vi "Named_Serial_Comms.vi"(0 "Channel Name":string, 1 "Write String":string, 2 "Timeout/ms":u32=500, 4 "!Error retries":i32=10, 6 "!Timeout retries":i32=3, 9 "Port Name":string, 11 "Term Grep":string="\r$", 12 "Log Errors?":bool=TRUE, 13 "Terminate Count":i32) -> (3 "Read":string="This is simulation mode", 10 "millisecond timer value":u32, 14 "Timed out":bool, 15 "Serial Error":bool)   [LabVIEW 2015]
doc: "The Serial Communication VI performs bidirectional communication with a port. It initializes the port, writes a string to the port, and performs a read with timeout. The Read with Timeout will wait until a terminating character is received or the time limit is up, whichever comes first.\nThe initialisation parameters, terminating character, and timeout, are all set in the Serial Setup Global."
uses:
  Port_Params.ctl
  <vilib>/Instr/_visa.llb/VISA Find Search Mode.ctl
  <vilib>/Instr/serial.llb/serpConfig.vi
panel:
  out "Buffer Trash":string
  out "Terminated?":bool
  out "Error Description":string
  in  "Uppercase?":bool
  in  "Append Return?":bool
  in  "Force setup reload":bool
  in  "Save Setups?":bool
  in  "!stop":bool
  out "byte count":u32
  out "Port Initialised?":bool[](array[boolean])
  out "Setting Number":i32
  out "Ports having file settings":string[](array[string])
  out "enumerated ports":string[](array[string])
  out "load setups error":bool
  out "Audit trail":string[](array[string])=["Start", "Simulate"]
  out "Close Port error":i32
  out "read error code":i32
  out "n-bytes error code":i32
  out "Write error":i32
  out "Port Initialisation Parameters":T1={"Name"="", "flow control etc."={"input XON/XOFF"=FALSE, "input HW Handshake"=FALSE, "input alt HW HShk"=FALSE, "output XON/XOFF"=FALSE, "output HW Handshake"=FALSE, "output alt HW HShk"=FALSE, "XOFF byte "=0, "XON byte"=0, "parity err byte"=0}, "buffer size"=0, "baud rate"=9600, "data bits"=8, "stop bits"=enum."1 bit", "parity"=enum."no parity"} {"flow control etc."."parity err byte" format="%.0x"; "flow control etc."."XON byte" format="%.0x"; "flow control etc."."XOFF byte" format="%.0x"; "data bits" min=5 max=8 step=1}
  out "Initialise error":i32
  out "Port Settings Array":T1[](array[typedef]) {"flow control etc."."parity err byte" format="%.0x"; "flow control etc."."XON byte" format="%.0x"; "flow control etc."."XOFF byte" format="%.0x"; "data bits" min=5 max=8 step=1}
  out "Case":string="Simulate"
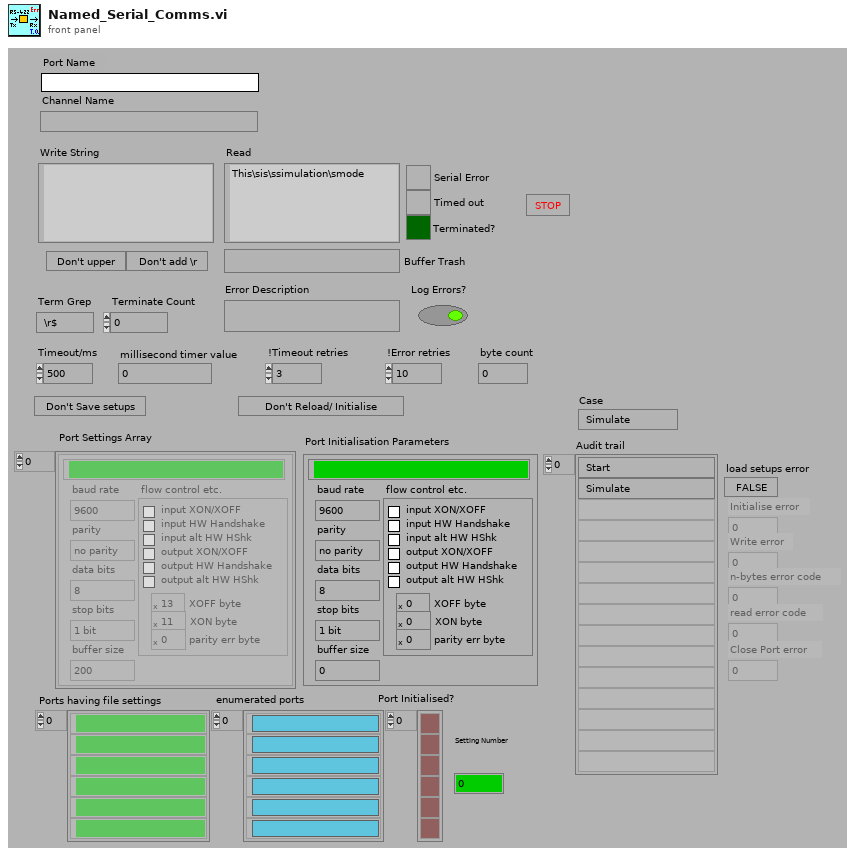
[diagram p1: front panel]
types:
  T1 = typedef "Port_Params.ctl" = cluster{"Name":string, "flow control etc.":cluster{"input XON/XOFF":bool, "input HW Handshake":bool, "input alt HW HShk":bool, "output XON/XOFF":bool, "output HW Handshake":bool, "output alt HW HShk":bool, "XOFF byte ":u8, "XON byte":u8, "parity err byte":u16}, "buffer size":u16, "baud rate":u32, "data bits":u16, "stop bits":enum16{"1 bit", "1.5 bits", "2 bits"}, "parity":enum16{"no parity", "odd parity", "even parity", "mark parity", "space parity"}}
  T2 = typedef "VISA Find Search Mode.ctl" = u32
  T3 = cluster{"input XON/XOFF":bool, "input HW Handshake":bool, "input alt HW HShk":bool, "output XON/XOFF":bool, "output HW Handshake":bool, "output alt HW HShk":bool, "XOFF byte ":u8, "XON byte":u8, "parity err byte":u16}
  T4 = enum16{"no parity", "odd parity", "even parity", "mark parity", "space parity"}
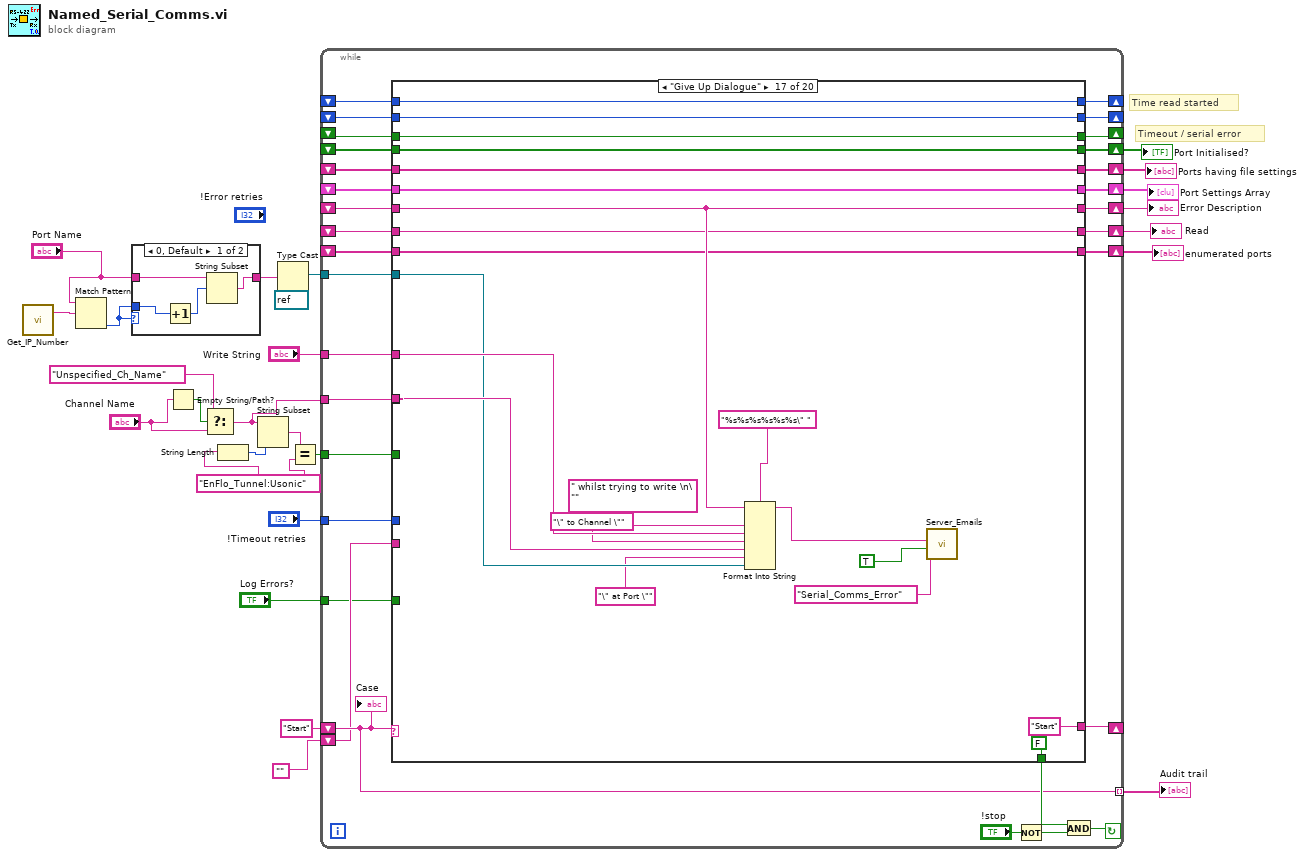
[diagram p0: block diagram]
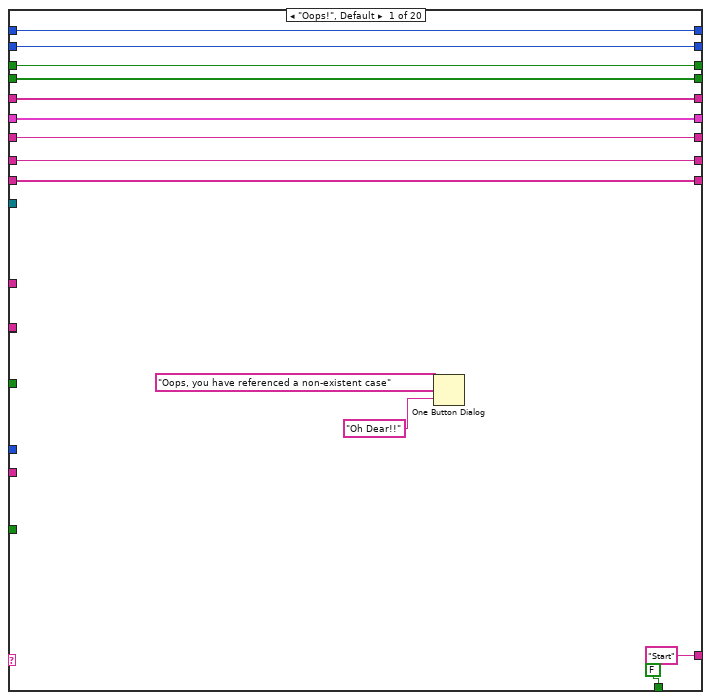
[diagram p3: hidden frame]
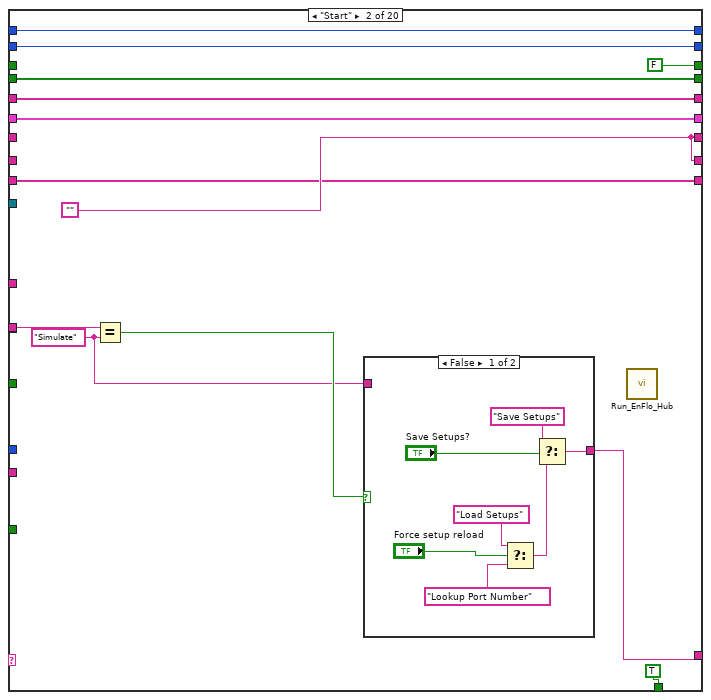
[diagram p4: hidden frame]
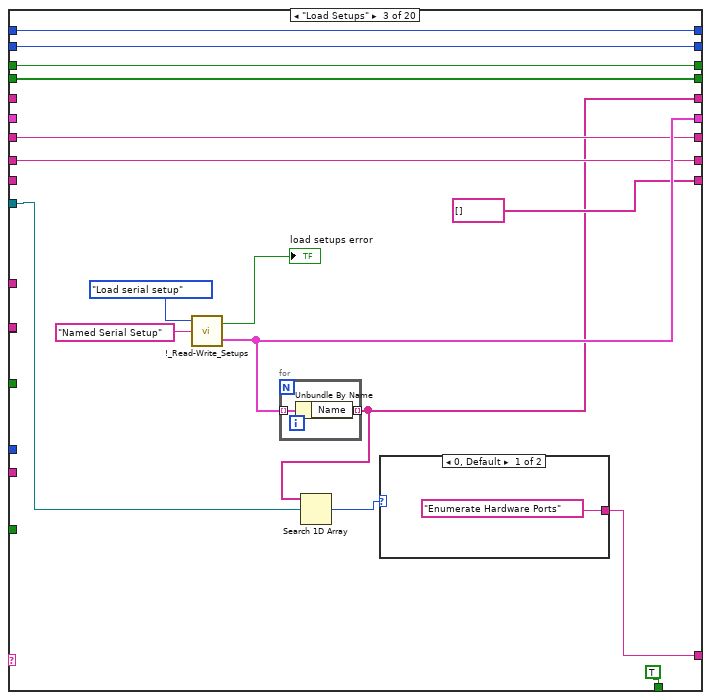
[diagram p6: hidden frame]
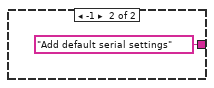
[diagram p7: hidden frame]
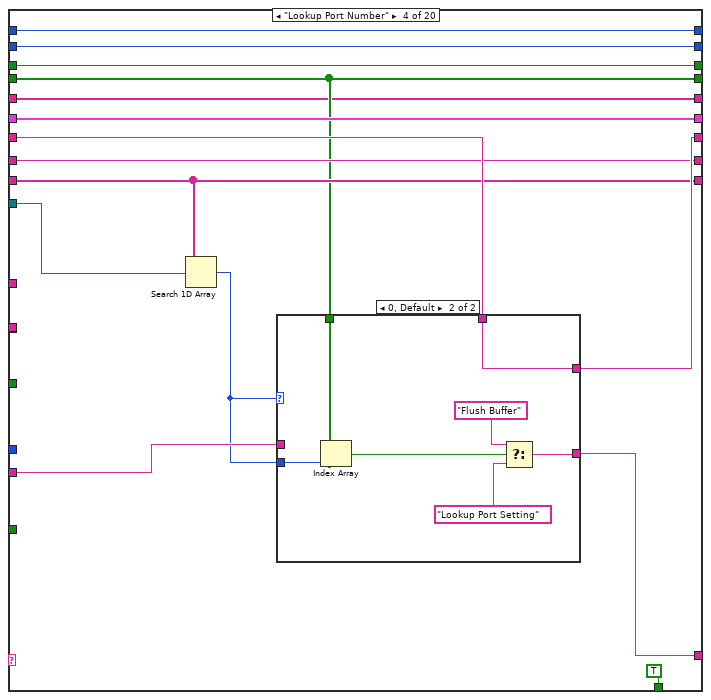
[diagram p8: hidden frame]
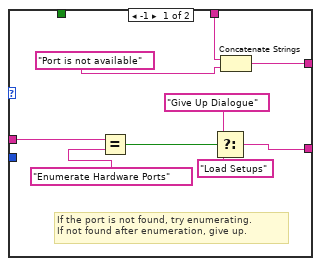
[diagram p9: hidden frame]
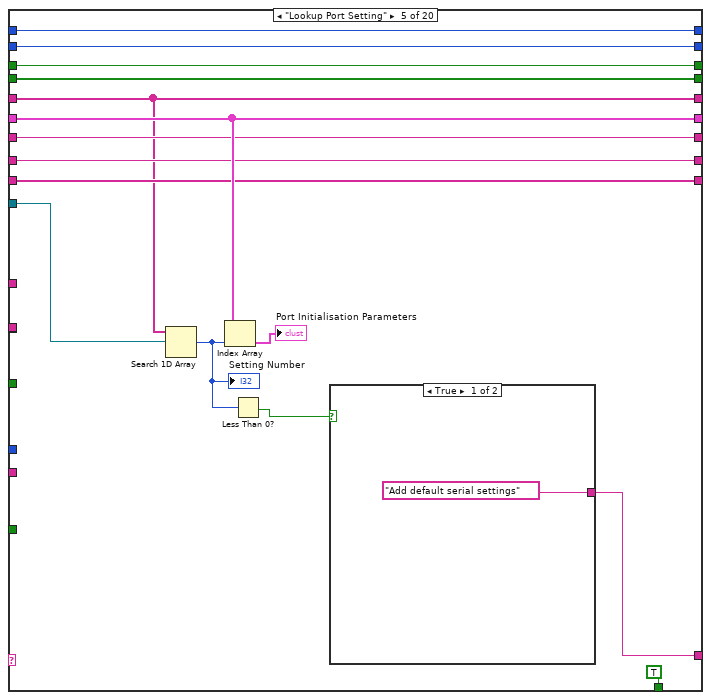
[diagram p10: hidden frame]
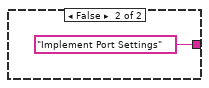
[diagram p11: hidden frame]
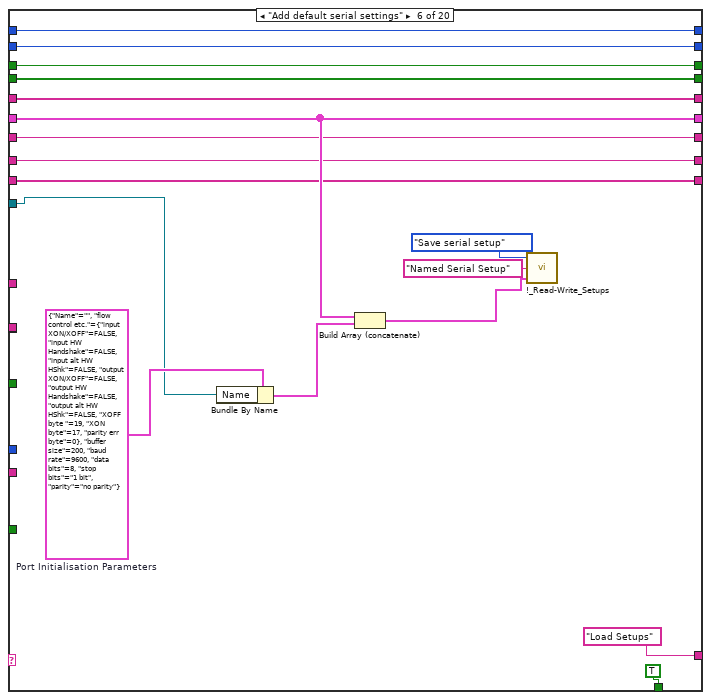
[diagram p12: hidden frame]
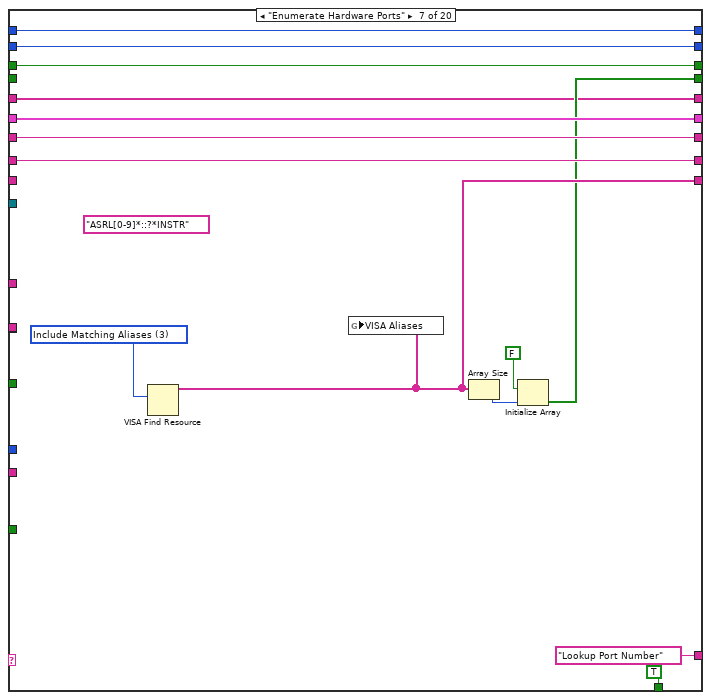
[diagram p13: hidden frame]
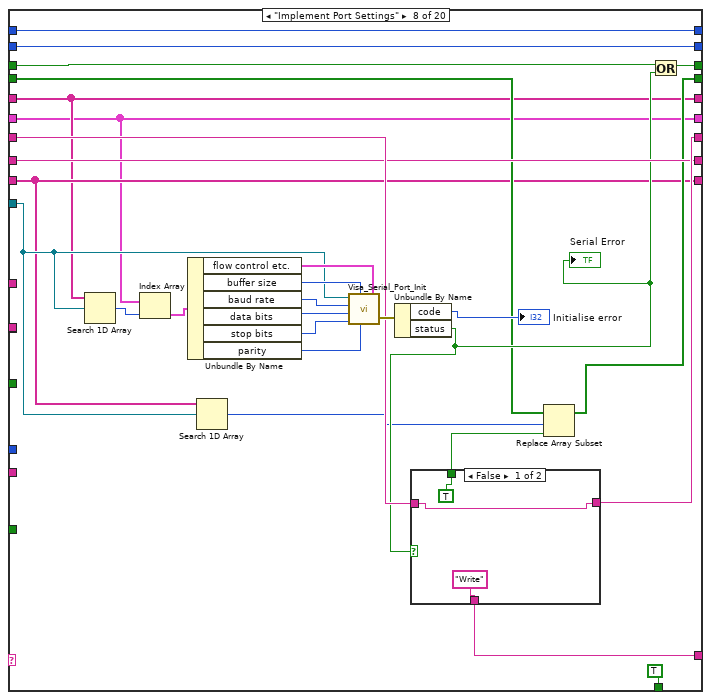
[diagram p14: hidden frame]
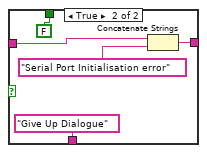
[diagram p15: hidden frame]
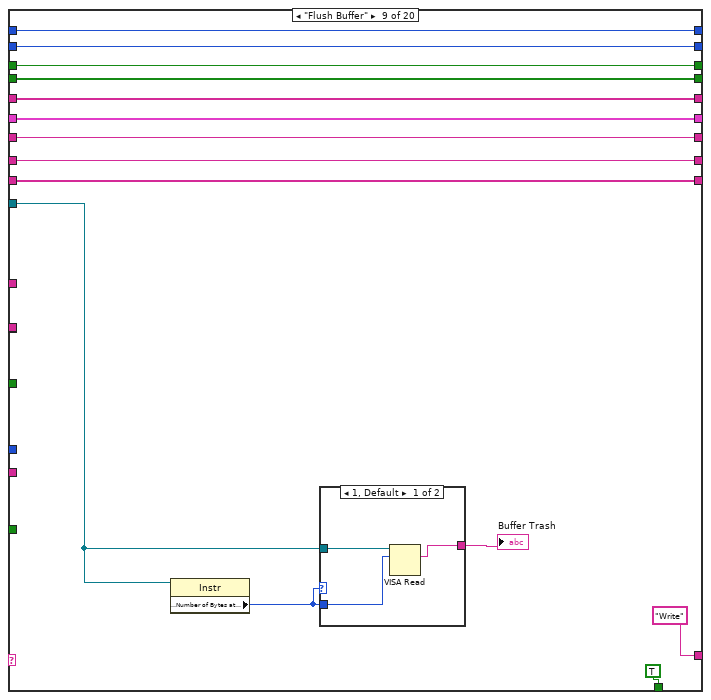
[diagram p16: hidden frame]
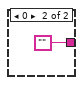
[diagram p17: hidden frame]
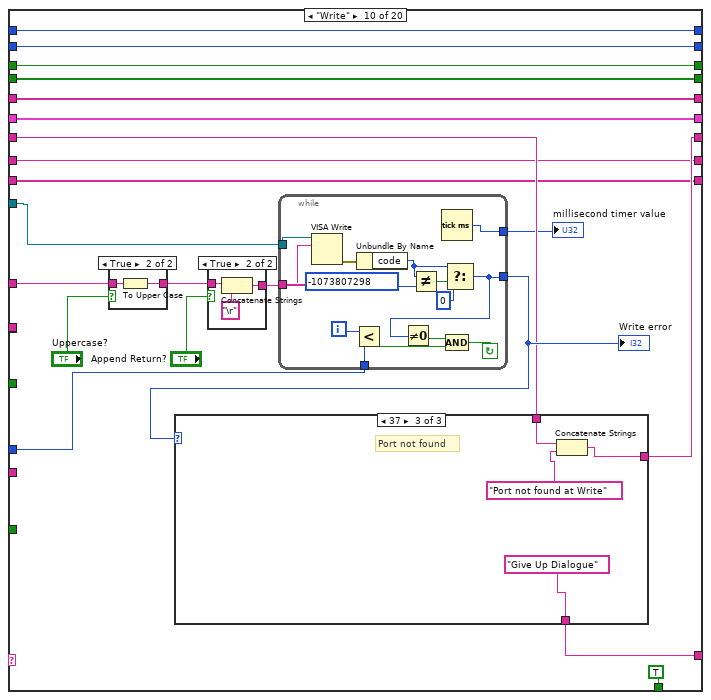
[diagram p18: hidden frame]
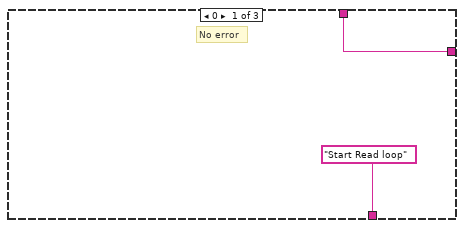
[diagram p19: hidden frame]
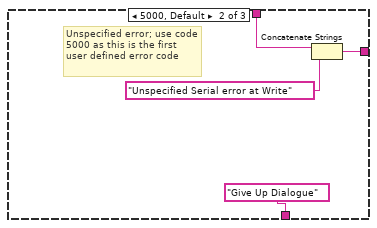
[diagram p20: hidden frame]
diagram:
  w19 = "EnFlo_Tunnel:Usonic"
  # "Time read started"
  # "Timeout / serial error"
  n1 = call "Get_IP_Number.vi"() -> ("IP Number"=w14:string)  [unwired: 1 out]
  n2 = Match Pattern(string="Port Name", regular expression=w14) -> (offset past match=w15:i32)  [unwired: 4 out]
  n3 = case shown="0, Default" w15 {
    tunnel: [w27 w31] -> w12
    tunnel: "Port Name" -> [w28 w31]
    tunnel: w15 -> [w30 _]
    frame 0, Default {
      n4 = Increment(x=w30) -> (x+1=w29:i32)
      n5 = String Subset(string=w28, offset (0)=w29) -> (substring=w27:string)  [unwired: 1 out]
    }
    frame -1 {
    }
  }
  n6 = Empty String/Path?(string/path="Channel Name") -> (empty?=w10:bool)
  n7 = Select(t="Unspecified_Ch_Name", s=w10, f="Channel Name") -> (s? t:f=w9:string)
  n8 = String Length(string=w19) -> (length=w21:i32)
  n9 = String Subset(string=w9, length (rest)=w21) -> (substring=w20:string)  [unwired: 1 out]
  n10 = Type Cast(type=refnum<visa-resource-name> refnum ("dup VISA resource name"), x=w12) -> (*(type *) &x=w17:refnum<visa-resource-name>)
  n11 = Equal?(x=w20, y=w19) -> (x = y?=w18:bool)
  n12 = while {
    tunnel: "!Timeout retries" -> [w52]
    tunnel: w9 -> [w54]
    shift-left: "" -> [w53]
    tunnel: [w55] -> w24 mode=indexing
    shift-left: "Start" -> [w55]
    shift-right: [w56] -> _
    tunnel: "Write String" -> [w61]
    tunnel: w17 -> [w62]
    tunnel: w18 -> [w51]
    tunnel: "Log Errors?" -> [w50]
    shift-right: [w49] -> w6
    shift-left: _ -> [w48]
    shift-right: [w46] -> w5
    shift-left: _ -> [w47]
    shift-right: [w45] -> w4
    shift-left: _ -> [w44]
    shift-right: [w43] -> w3
    shift-left: _ -> [w42]
    shift-right: [w41] -> _
    shift-left: _ -> [w40]
    shift-right: [w39] -> w2
    shift-left: _ -> [w38]
    shift-right: [w36] -> w1
    shift-left: _ -> [w37]
    shift-right: [w33] -> _
    shift-left: _ -> [w32]
    shift-right: [w35] -> _
    shift-left: _ -> [w34]
    stop <- w59 continue-if-true
    n13 = case shown="\"Give Up Dialogue\"" w55 {
      tunnel: w62 -> [_ _ w107 w131 w162 w179 _ w202 w238 w261 _ w322 w347 _ _ w440 w457 _ _ _]
      tunnel: w61 -> [_ _ _ _ _ _ _ _ _ w267 _ _ _ _ _ w433 w460 _ _ _]
      tunnel: ["Start" ("f") w88 w109 w129 w159 "Load Setups" ("f") "Lookup Port Number" w216 "Write" ("f") w264 "Bytes At Serial Port?" ("f") w324 w364 w387 w426 "Start" "Start" "Start" "Start" ("f") "Load Setups" ("f")] -> w56
      tunnel: [FALSE TRUE TRUE TRUE TRUE TRUE TRUE TRUE TRUE TRUE TRUE TRUE TRUE TRUE TRUE FALSE FALSE TRUE FALSE TRUE] -> w60
      tunnel: w54 -> [_ w86 _ _ _ _ _ _ _ _ _ _ _ _ _ w441 _ _ _ _]
      tunnel: w54 -> [_ _ _ _ _ _ _ _ _ _ _ _ _ _ _ _ w458 _ _ _]
      tunnel: w53 -> [_ _ _ w128 _ _ _ _ _ _ _ _ _ _ _ _ _ _ _ _]
      tunnel: w52 -> [_ _ _ _ _ _ _ _ _ w262 _ w323 _ _ _ _ _ _ _ _]
      tunnel: w51 -> [_ _ _ _ _ _ _ _ _ _ _ _ w360 _ _ _ _ _ _ _]
      tunnel: w50 -> [_ _ _ _ _ _ _ _ _ _ _ _ _ _ _ w439 _ _ _ _]
      tunnel: [w71 w83 w105 w127 w156 w173 w191 w199 w243 w260 w310 w321 w355 w380 w421 w438 w455 w473 w487 w498] -> w49
      tunnel: w48 -> [w71 w83 _ w127 w156 w173 w191 w199 w243 w260 w310 w321 w355 w380 w421 w438 w455 w473 w487 w498]
      tunnel: w47 -> [w70 _ w104 w126 w155 w172 w190 w211 w242 w258 w309 w320 w354 w379 w420 w437 w454 w472 w486 w497]
      tunnel: [w70 w82 w104 w125 w155 w172 w190 w212 w242 w259 w309 w320 w354 w379 w420 w437 w454 w472 w486 w497] -> w46
      tunnel: [w69 w82 w103 w124 w154 w171 w189 w210 w241 w257 "" w319 w353 w378 w419 w436 w453 w471 "Simulate" w496] -> w45
      tunnel: w44 -> [w69 _ w103 w124 w154 w171 w189 w210 w241 w257 _ w319 w352 w378 w419 w436 w453 w471 _ w496]
      tunnel: [w68 w81 string[] [] ("enumerated ports") w123 w153 w170 w188 w201 w240 w256 w307 w318 w351 w377 w418 w435 w452 w470 w484 w495] -> w43
      tunnel: w42 -> [w68 w81 _ w123 w153 w170 _ w201 w240 w256 w307 w318 w351 w377 w418 w435 w452 w470 w484 w495]
      tunnel: [w67 FALSE w101 w122 w152 w169 w187 w208 w236 w255 w306 w317 w350 w376 w416 w434 w451 w469 w483 w494] -> w41
      tunnel: w40 -> [w67 _ w101 w122 w152 w169 w187 w209 w236 w255 w306 w317 w350 w376 w417 w434 w451 w469 w483 w494]
      tunnel: [w66 w79 w100 w120 w151 w168 w186 w205 w235 w254 w305 w316 w349 w375 w414 w432 w450 w468 w482 w493] -> w39
      tunnel: w38 -> [w66 w79 w100 w120 w151 w168 _ w204 w235 w254 w305 w316 w349 w375 w414 w432 w450 w468 w482 w493]
      tunnel: [w65 w78 w99 w119 w150 w167 w185 w200 w234 w253 w304 w315 w348 w374 w413 w431 w449 w467 w481 w492] -> w36
      tunnel: w37 -> [w65 w78 _ w119 w150 w167 w185 w200 w234 w253 w304 w315 w348 w374 w413 w431 w449 w467 w481 w492]
      tunnel: [w64 w77 w98 w118 w149 w166 w184 w197 w233 w252 w303 w313 w343 w373 w412 w430 w448 w466 w480 w491] -> w35
      tunnel: w34 -> [w64 w77 w98 w118 w149 w166 w184 w197 w233 w252 _ w313 w343 w373 w412 w430 w448 w466 w480 w491]
      tunnel: [w63 w76 w97 w117 w148 w165 w183 w196 w232 w251 w302 w314 w342 w372 w411 w429 w447 w465 w479 w490] -> w33
      tunnel: w32 -> [w63 w76 w97 w117 w148 w165 w183 w196 w232 w251 w302 _ w342 w372 w411 w429 w447 w465 w479 w490]
      frame "Oops!", Default {
        n14 = One Button Dialog(message="Oops, you have referenced a non-existent case", button name ("OK")="Oh Dear!!") -> ()  [unwired: 1 out]
      }
      frame "Start" {
        w84 = "Simulate" ("y")
        w82 = ""
        n15 = Equal?(x=w86, y=w84) -> (x = y?=w85:bool)
        n16 = case shown="False" w85 {
          tunnel: [w91 w96] -> w88
          tunnel: w84 -> [_ w96]
          frame False {
            n17 = Select(t="Load Setups" ("f"), s="Force setup reload", f="Lookup Port Number") -> (s? t:f=w92:string)
            n18 = Select(t="Save Setups", s="Save Setups?", f=w92) -> (s? t:f=w91:string)
          }
          frame True {
          }
        }
        n19 = call "Run_EnFlo_Hub.vi"() -> ()  [unwired: 8 out]
      }
      frame "Load Setups" {
        n20 = call "!_Read-Write_Setups.vi"("Setup Name"="Named Serial Setup", "Mode"=enum16{"Load serial setup", "Save serial setup"}."Load serial setup") -> ("Port Settings Array Out"=w105:T1[], "error unflattening"=→"load setups error":bool)  [unwired: 1 in]
        n21 = for {
          tunnel: w105 -> [w116] mode=indexing
          tunnel: [w115] -> w99 mode=indexing
          n22 = Unbundle By Name(w116) -> ("Name"=w115:string)
        }
        n23 = Search 1D Array(1D array=w99, element=w107) -> (index of element=w106:i32)  [unwired: 1 out]
        n24 = case shown="0, Default" w106 {
          tunnel: ["Enumerate Hardware Ports" "Add default serial settings"] -> w109
          frame 0, Default {
          }
          frame -1 {
          }
        }
      }
      frame "Lookup Port Number" {
        n25 = Search 1D Array(1D array=w123, element=w131) -> (index of element=w121:i32)  [unwired: 1 out]
        n26 = case shown="0, Default" w121 {
          tunnel: [w140 w147] -> w129
          tunnel: w121 -> [_ w146]
          tunnel: w128 -> [w137 _]
          tunnel: w126 -> [w133 w142]
          tunnel: [w132 w142] -> w125
          tunnel: w120 -> [_ w141]
          frame -1 {
            # "If the port is not found, try enumerating.\nIf not found after enumeration, give up."
            n27 = Equal?(x=w137, y="Enumerate Hardware Ports" ("f")) -> (x = y?=w139:bool)
            n28 = Select(t="Give Up Dialogue" ("f"), s=w139, f="Load Setups") -> (s? t:f=w140:string)
            n29 = Concatenate Strings(w133, "Port is not available" ("Error Description")) -> (w132:string)
          }
          frame 0, Default {
            n30 = Index Array(array=w141, index=w146) -> (element=w145:bool)
            n31 = Select(t="Flush Buffer" ("f"), s=w145, f="Lookup Port Setting") -> (s? t:f=w147:string)
          }
        }
      }
      frame "Lookup Port Setting" {
        n32 = Search 1D Array(1D array=w150, element=w162) -> (index of element=w158:i32)  [unwired: 1 out]
        "Setting Number" <- w158
        n33 = Index Array(array=w156, index=w158) -> (element=→"Port Initialisation Parameters":T1)
        n34 = Less Than 0?(x=w158) -> (x < 0?=w157:bool)
        n35 = case shown="True" w157 {
          tunnel: ["Add default serial settings" "Implement Port Settings"] -> w159
          frame True {
          }
          frame False {
          }
        }
      }
      frame "Add default serial settings" {
        w181 = T1 {"Name"="", "flow control etc."={"input XON/XOFF"=FALSE, "input HW Handshake"=FALSE, "input alt HW HShk"=FALSE, "output XON/XOFF"=FALSE, "output HW Handshake"=FALSE, "output alt HW HShk"=FALSE, "XOFF byte "=19, "XON byte"=17, "parity err byte"=0}, "buffer size"=200, "baud rate"=9600, "data bits"=8, "stop bits"=enum."1 bit", "parity"=enum."no parity"}  # Port Initialisation Parameters
        n36 = Bundle By Name(cluster=w181, "Name"=w179) -> (w180:T1)
        n37 = Build Array (concatenate)(w173, w180) -> (w176:T1[])
        n38 = call "!_Read-Write_Setups.vi"("Port Settings Array In"=w176, "Setup Name"="Named Serial Setup", "Mode"=enum16{"Load serial setup", "Save serial setup"}."Save serial setup") -> ()  [unwired: 2 out]
      }
      frame "Enumerate Hardware Ports" {
        w182 = T2 3 items=["Canonical Names Only"=0, "Aliases Only"=2, "Include Matching Aliases"=3, "Include All Aliases"=4] ("Search Mode")
        (unwired) "ASRL[0-9]*::?*INSTR" ("expression (\"?*\")")
        n39 = VISA Find Resource(10:w182) -> (3:w188:string[])  [unwired: 1 in, 3 out]
        n40 = global write "serpConfig.vi" "VISA Aliases"(w188) -> ()
        n41 = Array Size(array=w188) -> (size(s)=w193:i32)
        n42 = Initialize Array(FALSE, w193) -> (w186:bool[])
      }
      frame "Implement Port Settings" {
        n43 = Search 1D Array(1D array=w200, element=w202) -> (index of element=w203:i32)  [unwired: 1 out]
        n44 = Index Array(array=w199, index=w203) -> (element=w198:T1)
        n45 = Unbundle By Name(w198) -> ("flow control etc."=w223:T3, "buffer size"=w222:u16, "baud rate"=w221:u32, "data bits"=w220:u16, "stop bits"=w219:enum16{"1 bit", "1.5 bits", "2 bits"}, "parity"=w218:T4)
        n46 = Search 1D Array(1D array=w201, element=w202) -> (index of element=w206:i32)  [unwired: 1 out]
        n47 = call "Visa_Serial_Port_Init.vi"("flow control etc."=w223, "parity"=w218, "buffer size"=w222, "stop bits"=w219, "data bits"=w220, "baud rate"=w221, "Visa Port Name"=w202) -> ("error out"=w214:errorcluster)
        n48 = Unbundle By Name(w214) -> ("code"=→"Initialise error":i32, "status"=w207:bool)
        "Serial Error" <- w207
        n49 = case shown="False" w207 {
          tunnel: ["Write" "Give Up Dialogue"] -> w216
          tunnel: [TRUE ("Element Data") FALSE ("Element Data")] -> w215
          tunnel: [w224 w228] -> w212
          tunnel: w211 -> [w224 w227]
          frame False {
          }
          frame True {
            n50 = Concatenate Strings(w227, "Serial Port Initialisation error" ("Error Description")) -> (w228:string)
          }
        }
        n51 = Replace Array Subset(array=w204, new element=w215, index=w206) -> (w205:bool[])
        n52 = Or(x=w209, y=w207) -> (x .or. y?=w208:bool)
      }
      frame "Flush Buffer" {
        n53 = property class="Instr"(reference=w238) -> ("Serial Settings:Number of Bytes at Serial Port"=w239:u32)  [unwired: 1 in, 2 out]
        n54 = case shown="1, Default" w239 {
          tunnel: [w248 ""] -> w237
          tunnel: w238 -> [w247 _]
          tunnel: w239 -> [w246 _]
          frame 1, Default {
            n55 = VISA Read(VISA resource name=w247, byte count=w246) -> (read buffer=w248:string)  [unwired: 1 in, 3 out]
          }
          frame 0 {
          }
        }
        "Buffer Trash" <- w237
      }
      frame "Write" {
        n56 = case shown="True" "Uppercase?" {
          tunnel: w267 -> [w299 w301]
          tunnel: [w299 w300] -> w269
          frame False {
          }
          frame True {
            n57 = To Upper Case(1:w301) -> (0:w300:string)
          }
        }
        n58 = case shown="True" "Append Return?" {
          tunnel: w269 -> [w295 w298]
          tunnel: [w295 w297] -> w266
          frame False {
          }
          frame True {
            n59 = Concatenate Strings(w298, "\r") -> (w297:string)
          }
        }
        n60 = while {
          tunnel: w262 -> [w280]
          tunnel: [w271] -> w263
          tunnel: w266 -> [w278]
          tunnel: w261 -> [w277]
          tunnel: [w276] -> w250
          i -> [w284]
          stop <- w281 continue-if-true
          n61 = VISA Write(VISA resource name=w277, write buffer=w278) -> (error out=w279:errorcluster)  [unwired: 1 in, 2 out]
          n62 = Less?(x=w284, y=w280) -> (x < y?=w283:bool)
          n63 = Unbundle By Name(w279) -> ("code"=w273:i32)
          n64 = Not Equal?(x=w273, y=-1073807298 ("code")) -> (x != y?=w274:bool)
          n65 = Tick Count (ms)() -> (millisecond timer value=w276:u32)
          n66 = Select(t=w273, s=w274, f=0) -> (s? t:f=w271:i32)
          n67 = Not Equal To 0?(x=w271) -> (x != 0?=w282:bool)
          n68 = Compound Arithmetic op=AND(w282, w283) -> (w281:bool)
        }
        "Write error" <- w263
        "millisecond timer value" <- w250
        n69 = case shown="37" w263 {
          tunnel: ["Start Read loop" "Give Up Dialogue" "Give Up Dialogue"] -> w264
          tunnel: [w285 w288 w291] -> w259
          tunnel: w258 -> [w285 w287 w293]
          frame 0 {
            # "No error"
          }
          frame 5000, Default {
            # "Unspecified error; use code 5000 as this is the first user defined error code"
            n70 = Concatenate Strings(w287, "Unspecified Serial error at Write" ("Error Description")) -> (w288:string)
          }
          frame 37 {
            # "Port not found"
            n71 = Concatenate Strings(w293, "Port not found at Write" ("Error Description")) -> (w291:string)
          }
        }
      }
      frame "Start Read loop" {
        n72 = Tick Count (ms)() -> (millisecond timer value=w303:u32)
      }
      frame "Bytes At Serial Port?" {
        n73 = while {
          tunnel: w323 -> [w333]
          tunnel: [w330] -> w314
          tunnel: [w334] -> w327
          tunnel: w322 -> [w331]
          i -> [w337]
          stop <- w335 continue-if-true
          n74 = property class="Instr"(reference=w331) -> (error out=w329:errorcluster, "Serial Settings:Number of Bytes at Serial Port"=w330:u32)  [unwired: 1 in, 1 out]
          "byte count" <- w330
          n75 = Unbundle By Name(w329) -> ("code"=w332:i32)
          "n-bytes error code" <- w332
          n76 = Less?(x=w337, y=w333) -> (x < y?=w336:bool)
          n77 = Equal To 0?(x=w332) -> (x = 0?=w334:bool)
          n78 = Compound Arithmetic op=AND(invert w334, w336) -> (w335:bool)
          n79 = case shown="False" w335 {
            frame False {
            }
            frame True {
              n80 = Wait (ms)(milliseconds to wait=u32 5) -> ()  [unwired: 1 out]
            }
          }
        }
        n81 = case shown="1, Default" w314 {
          tunnel: ["Serial Port Read" ("f") "Check for Termination" ("f")] -> w325
          frame 1, Default {
          }
          frame 0 {
            n82 = Wait (ms)(milliseconds to wait=u32 1) -> ()  [unwired: 1 out]
          }
        }
        n83 = Select(t=w325, s=w327, f="Log") -> (s? t:f=w324:string)
      }
      frame "Serial Port Read" {
        n84 = Greater?(x=w342, y=u32 1) -> (0:w359:bool)
        n85 = And(x=w359, y=w360) -> (x .and. y?=w358:bool)
        n86 = case shown="True" w358 {
          tunnel: w342 -> [w369 w371]
          tunnel: [w369 w370] -> w344
          frame False {
          }
          frame True {
            n87 = Decrement(x=w371) -> (x-1=w370:u32)
          }
        }
        n88 = VISA Read(VISA resource name=w347, byte count=w344) -> (read buffer=w345:string, error out=w346:errorcluster)  [unwired: 1 in, 2 out]
        n89 = Unbundle By Name(w346) -> ("code"=w357:i32)
        n90 = case shown="0, Default" w357 {
          selector: w357 -> [w367 _]
          tunnel: [w367 0 ("code")] -> w356
          frame 0, Default {
          }
          frame 1073676294 {
          }
        }
        "read error code" <- w356
        n91 = Concatenate Strings(w352, w345) -> (w353:string)
        n92 = Equal To 0?(x=w356) -> (x = 0?=w363:bool)
        n93 = Select(t="Check for Termination" ("f"), s=w363, f="Log") -> (s? t:f=w364:string)
      }
      frame "Check for Termination" {
        n94 = Empty String/Path?(string/path="Term Grep") -> (empty?=w389:bool)
        n95 = case shown="False" w389 {
          tunnel: "Terminate Count" -> [w393 w408]
          tunnel: w378 -> [w395 w409]
          tunnel: [w390 w407] -> w384
          tunnel: "Term Grep" -> [w396 _]
          frame False {
            n96 = Decrement(x=w393) -> (x-1=w392:i32)
            n97 = while {
              tunnel: [w397] -> w391
              tunnel: w392 -> [w400]
              shift-left: 0 -> [w404]
              shift-right: [w403] -> _
              tunnel: w395 -> [w405]
              tunnel: w396 -> [w406]
              i -> [w401]
              stop <- w398 continue-if-true
              n98 = Match Pattern(string=w405, regular expression=w406, offset (0)=w404) -> (match substring=w397:string, offset past match=w403:i32)  [unwired: 2 out]
              n99 = Less?(x=w401, y=w400) -> (x < y?=w399:bool)
              n100 = Greater Or Equal To 0?(x=w403) -> (x >= 0?=w402:bool)
              n101 = Compound Arithmetic op=AND(w402, w399) -> (w398:bool)
            }
            n102 = Empty String/Path?(string/path=w391) -> (empty?=w390:bool)
          }
          frame True {
            n103 = String Length(string=w409) -> (length=w410:i32)
            n104 = Less?(x=w410, y=w408) -> (x < y?=w407:bool)
          }
        }
        n105 = Not(x=w384) -> (.not. x?=w381:bool)
        "Terminated?" <- w381
        n106 = Select(t="Log" ("f"), s=w381, f="TimeOut?") -> (s? t:f=w387:string)
      }
      frame "TimeOut?" {
        n107 = Tick Count (ms)() -> (millisecond timer value=w427:u32)
        n108 = Subtract(x=w427, y=w412) -> (x-y=w428:u32)
        n109 = Greater?(x=w428, y="Timeout/ms") -> (0:w415:bool)
        "Timed out" <- w415
        n110 = Select(t="Log" ("f"), s=w415, f="Bytes At Serial Port?") -> (s? t:f=w426:string)
        n111 = Or(x=w417, y=w415) -> (x .or. y?=w416:bool)
      }
      frame "Log" {
        n112 = call "!_Serial_log_builder.vi"("Port Name"=w440, "Comms Error"=w434, "Channel Name"=w441, "Write String"=w433, "Log Errors?"=w439, "Read"=w436) -> ()  [unwired: 3 out]
      }
      frame "Give Up Dialogue" {
        n113 = Format Into String(format string="%s%s%s%s%s%s\" ", initial string=w454, " whilst trying to write \n\"", w460, "\" to Channel \"", w458, "\" at Port \"" ("Input 5"), w457) -> (resulting string=w446:string)  [unwired: 1 in, 1 out]
        n114 = call "Server_Emails.vi"("Message"=w446, "Contact All clients?"=TRUE, "Subject"="Serial_Comms_Error") -> ()  [unwired: 2 in, 3 out]
      }
      frame "Close All Ports" {
        n115 = for {
          tunnel: w470 -> [w476] mode=indexing
          n116 = VISA Close(VISA resource name=w476) -> (error out=w478:errorcluster)  [unwired: 1 in]
          n117 = Unbundle By Name(w478) -> ("code"=→"Close Port error":i32)
        }
      }
      frame "Simulate" {
        (unwired) "This is simulation mode" ("Read")
      }
      frame "Save Setups" {
        n118 = call "!_Read-Write_Setups.vi"("Port Settings Array In"=w498, "Setup Name"="Named Serial Setup", "Mode"=enum16{"Load serial setup", "Save serial setup"}."Save serial setup") -> ()  [unwired: 2 out]
      }
    }
    n119 = Not(x="!stop") -> (.not. x?=w57:bool)
    n120 = And(x=w60, y=w57) -> (x .and. y?=w59:bool)
    "Case" <- w55
  }
  "Audit trail" <- w24
  "Port Settings Array" <- w6
  "Error Description" <- w5
  "Read" <- w4
  "enumerated ports" <- w3
  "Port Initialised?" <- w2
  "Ports having file settings" <- w1
